vi "Net DC Min Max Mean.vi"(0 "Positive Pulses - Passive":dbl[](array[numeric]), 1 "Negative Pulses - Passive":dbl[](array[numeric]), 2 "Positive Pulses - Active":dbl[](array[numeric]), 3 "Negative Pulses - Active":dbl[](array[numeric])) -> (5 "Min":dbl, 6 "Max":dbl, 7 "Mean":dbl)   [LabVIEW 2010]
uses:
  <vilib>/Analysis/NI_AALBase.lvlib
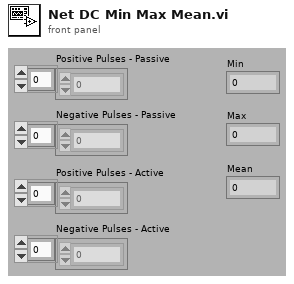
[diagram p1: front panel]
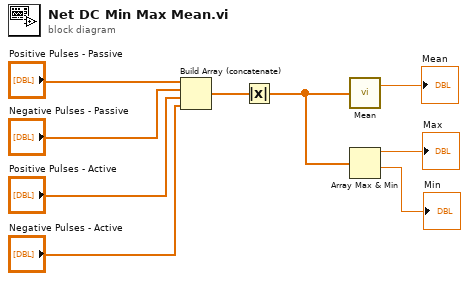
[diagram p0: block diagram]
diagram:
  n1 = Build Array (concatenate)("Positive Pulses - Passive", "Negative Pulses - Passive", "Positive Pulses - Active", "Negative Pulses - Active") -> (w7:dbl[])
  n2 = Absolute Value(x=w7) -> (abs(x)=w5:dbl[])
  n3 = call <vilib>:"Mean.vi"("X"=w5) -> ("mean"=→"Mean":dbl)  [unwired: 1 out]
  n4 = Array Max & Min(array=w5) -> (max value=→"Max":dbl, min value=→"Min":dbl)  [unwired: 2 out]
